vi "Set-Query SESER.vi"(8 "error in (no error)":errorcluster {"code" format="%.0x"}, 9 "Enable SESER":T2, 10 "Enable Mask (T)":bool=TRUE, 11 "VISA session":refnum<visa-resource-name>) -> (0 "error out":errorcluster {"code" format="%.0x"}, 1 "Read SESER":T1, 3 "dup VISA session":refnum<visa-resource-name>)   [LabVIEW 2011]
doc: "Sets or queries the bits in the instrument's IEEE-488.2 Standard Event Status Enable Register (SESER). \n\nNote: Reading the SESER reads the current mask status. To read the actual value\nof the Standard Event Status Register (SESR), call the Query SESR.vi"
uses:
  Low Level/Standadard Event Status Enable Control.ctl
  Low Level/Standard Event Status Indicator.ctl
panel:
  # "standard event status enable register (SESER)"
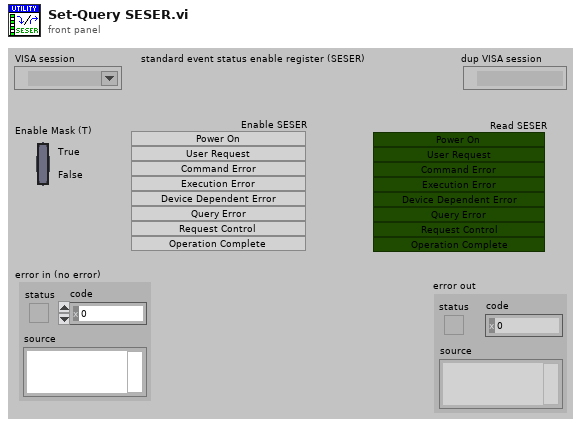
[diagram p1: front panel]
types:
  T1 = typedef "Standard Event Status Indicator.ctl" = cluster{"Operation Complete (1)":bool, "Request Control (2)":bool, "Query Error (4)":bool, "Device Dependent Error (8)":bool, "Execution Error (16)":bool, "Command Error (32)":bool, "User Request (64)":bool, "Power On (128)":bool}
  T2 = typedef "Standadard Event Status Enable Control.ctl" = cluster{"Operation Complete (1)":bool, "Request Control (2)":bool, "Query Error (4)":bool, "Device Dependent Error (8)":bool, "Execution Error (16)":bool, "Command Error (32)":bool, "User Request (64)":bool, "Power On (128)":bool}
  T3 = cluster{"[0]":bool, "[1]":bool, "[2]":bool, "[3]":bool, "[4]":bool, "[5]":bool, "[6]":bool, "[7]":bool}
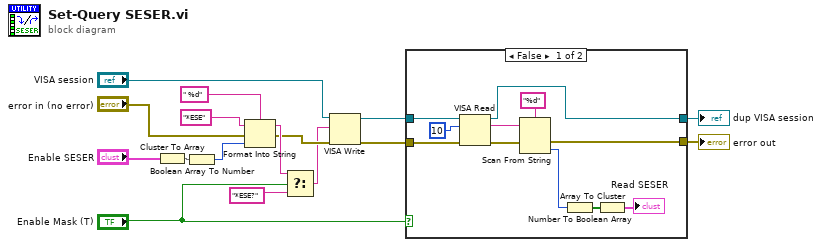
[diagram p0: block diagram]
diagram:
  n1 = Cluster To Array(cluster="Enable SESER") -> (array=w16:bool[])
  n2 = Boolean Array To Number(Boolean array=w16) -> (number=w11:u32)
  n3 = Format Into String(format string=" %d", initial string="*ESE", error in="error in (no error)", w11) -> (resulting string=w9:string, error out=w8:errorcluster)
  n4 = Select(t=w9, s="Enable Mask (T)", f="*ESE?") -> (s? t:f=w7:string)
  n5 = VISA Write(VISA resource name="VISA session", write buffer=w7, error in (no error)=w8) -> (VISA resource name out=w14:refnum<visa-resource-name>, error out=w15:errorcluster)  [unwired: 1 out]
  n6 = case shown="False" "Enable Mask (T)" {
    tunnel: w15 -> [w24 w29]
    tunnel: w14 -> [w25 w28]
    tunnel: [w18 w29] -> w5
    tunnel: [w17 w28] -> w6
    frame False {
      n7 = VISA Read(VISA resource name=w25, byte count=10, error in (no error)=w24) -> (VISA resource name out=w17:refnum<visa-resource-name>, read buffer=w21:string, error out=w19:errorcluster)  [unwired: 1 out]
      n8 = Scan From String(format string="%d", input string=w21, error in=w19) -> (error out=w18:errorcluster, output 1=w20:i32)  [unwired: 2 in, 2 out]
      n9 = Number To Boolean Array(number=w20) -> (Boolean array=w27:bool[])
      n10 = Array To Cluster(array=w27) -> (cluster=→"Read SESER":T3)
    }
    frame True {
    }
  }
  "error out" <- w5
  "dup VISA session" <- w6
